vi "czas.vi"(1 "czas":dbl) -> (0 "czas jaki upłynął":dbl)   [LabVIEW 2018]
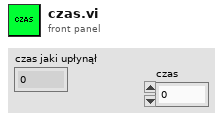
[diagram p1: front panel]
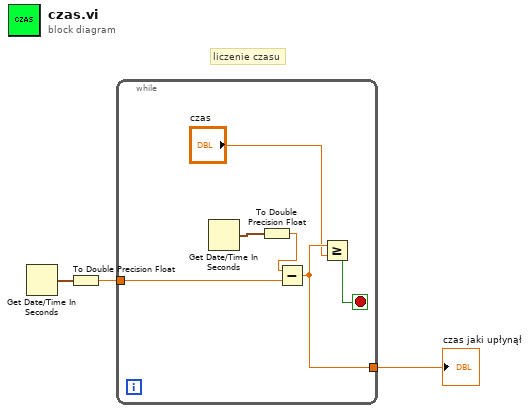
[diagram p0: block diagram]
diagram:
  # "liczenie czasu"
  n1 = Get Date/Time In Seconds() -> (seconds since 1Jan1904=w3:timestamp)
  n2 = To Double Precision Float(number=w3) -> (double precision float=w2:dbl)
  n3 = while {
    tunnel: w2 -> [w7]
    tunnel: [w5] -> w1
    stop <- w6 stop-if-true
    n4 = Get Date/Time In Seconds() -> (seconds since 1Jan1904=w9:timestamp)
    n5 = To Double Precision Float(number=w9) -> (double precision float=w8:dbl)
    n6 = Subtract(x=w8, y=w7) -> (x-y=w5:dbl)
    n7 = Greater Or Equal?(x=w5, y="czas") -> (x >= y?=w6:bool)
  }
  "czas jaki upłynął" <- w1
